vi "NMT send.vi"(4 "error in (no error)":errorcluster, 5 "Node ID":u8, 6 "Command specifier":u8(ring)=1 items=["Start remote node"=1, "Stop remote node"=2, "Enter pre-operational state"=128, "Reset node"=129, "Reset communication"=130], 7 "CANopen in":refnum<class "CANopen.lvclass">) -> (0 "error out":errorcluster, 3 "CANopen out":refnum<class "CANopen.lvclass">)   [LabVIEW 2024, in "canopen.lvlib" / "CANopen.lvclass"]
doc: "Sends a NMT message. If \"Node ID\" is not specified, the message will be broadcasted."
uses:
  CANopen.lvclass
  FunctionCode.ctl
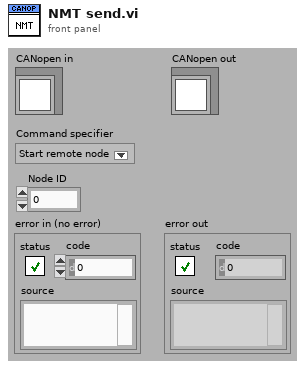
[diagram p1: front panel]
types:
  T1 = typedef "canopen.lvlib/CANopen.lvclass/FunctionCode.ctl" = u8
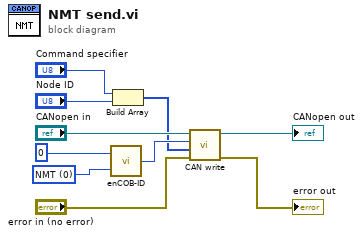
[diagram p0: block diagram]
diagram:
  w3 = T1 0 items=["NMT", "SYNC", "TIME STAMP", "EMERGENCY", "PDO1 (tx)", "PDO1 (rx)", "PDO2 (tx)", "PDO2 (rx)", "PDO3 (tx)", "PDO3 (rx)", "PDO4 (tx)", "PDO4 (rx)", "SDO (tx)", "SDO (rx)", "NMT Error Control"] ("Function code")
  n1 = call "enCOB-ID.vi"("Function code"=w3, "Node ID"=u16 0) -> ("Cob ID"=w2:u32)
  n2 = Build Array("Command specifier", "Node ID") -> (w1:u8[])
  n3 = call "CAN write.vi"("error in (no error)"="error in (no error)", "Data"=w1, "COB id"=w2, "CANopen in"="CANopen in") -> ("error out"=→"error out":errorcluster, "CANopen out"=→"CANopen out":refnum<class "CANopen.lvclass">)  [unwired: 1 in, 1 out]
